vi "Day 2 - Red-Nosed Reports.vi"() -> ()   [LabVIEW 2020, in "AoC 2024.lvlib"]
uses:
  AoC 2024.lvlib
panel:
  out "Puzzle Part-2 Answer":string
  out "Puzzle Answer":string
  in  "Puzzle Input":string="7 6 4 2 1\n1 2 7 8 9\n9 7 6 2 1\n1 3 2 4 5\n8 6 4 4 1\n1 3 6 7 9"
  # "Enter the Puzzle Input and run the VI"
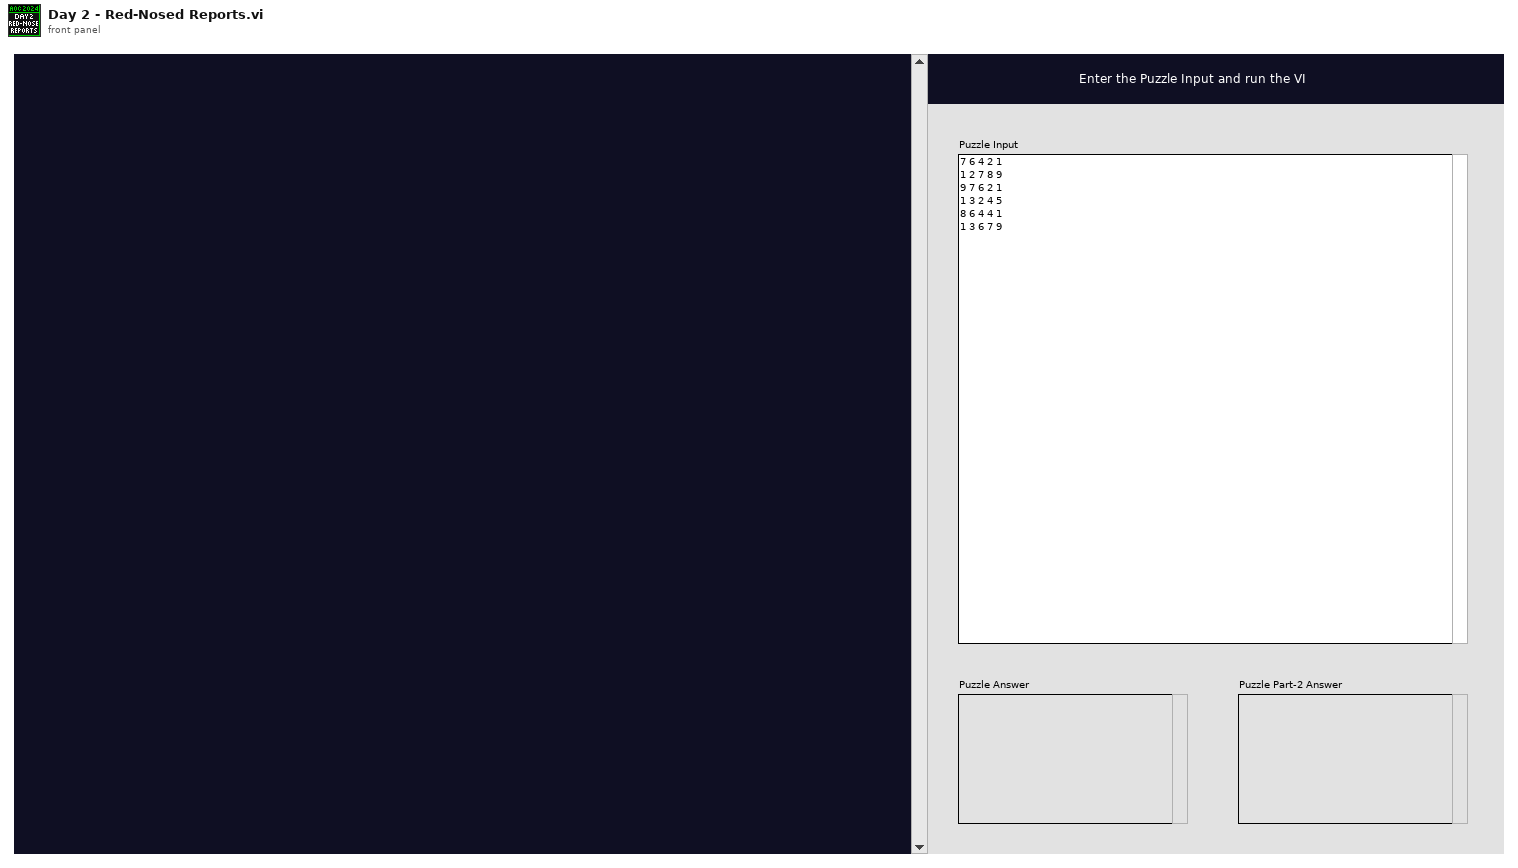
[diagram p1: front panel]
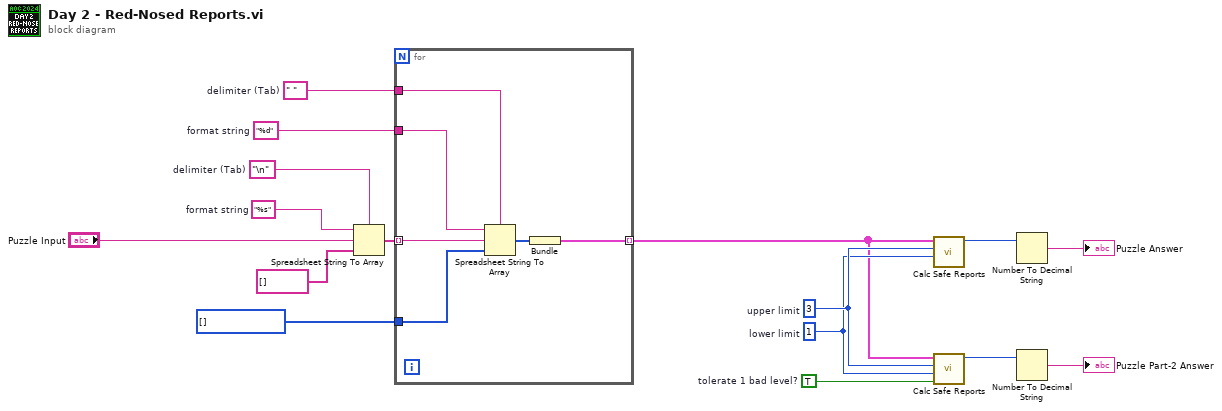
[diagram p0: block diagram]
diagram:
  w1 = TRUE  # tolerate 1 bad level?
  w4 = "%d"  # format string
  w6 = " "  # delimiter (Tab)
  w10 = 1  # lower limit
  w11 = 3  # upper limit
  w12 = "\n"  # delimiter (Tab)
  w13 = "%s"  # format string
  n1 = Spreadsheet String To Array(delimiter (Tab)=w12, format string=w13, spreadsheet string="Puzzle Input", array type (2D Dbl)=string[] []) -> (array=w3:string[])
  n2 = for {
    tunnel: w6 -> [w22]
    tunnel: i32[] [] -> [w21]
    tunnel: w4 -> [w19]
    tunnel: w3 -> [w18] mode=indexing
    tunnel: [w17] -> w2 mode=indexing
    n3 = Spreadsheet String To Array(delimiter (Tab)=w22, format string=w19, spreadsheet string=w18, array type (2D Dbl)=w21) -> (array=w20:i32[])
    n4 = Bundle(w20) -> (w17:cluster{i32[]})  [unwired: 1 in]
  }
  n5 = call "Calc Safe Reports.vi"("lower limit"=w10, "upper limit"=w11, "Reports"=w2) -> ("safe reports"=w8:u32)  [unwired: 8 in]
  n6 = call "Calc Safe Reports.vi"("tolerate 1 bad level?"=w1, "lower limit"=w10, "upper limit"=w11, "Reports"=w2) -> ("safe reports"=w9:u32)  [unwired: 7 in]
  n7 = Number To Decimal String(number=w8) -> (decimal integer string=→"Puzzle Answer":string)  [unwired: 1 in]
  n8 = Number To Decimal String(number=w9) -> (decimal integer string=→"Puzzle Part-2 Answer":string)  [unwired: 1 in]
